vi "FTW-Endpoint-TCP-Connection-Get.vi"(8 "error in (no error)":errorcluster, 11 "FTW-Endpoint-TCP in":refnum<class "FTW-Endpoint-TCP.lvclass">) -> (0 "error out":errorcluster, 2 "Connection":refnum<k5>, 3 "FTW-Endpoint-TCP out":refnum<class "FTW-Endpoint-TCP.lvclass">)   [LabVIEW 2015, in "FTW-Endpoint-TCP.lvclass"]
uses:
  FTW-Endpoint-TCP.lvclass
  FTW-Endpoint-TCP.lvclass/FTW-Endpoint-TCP.ctl
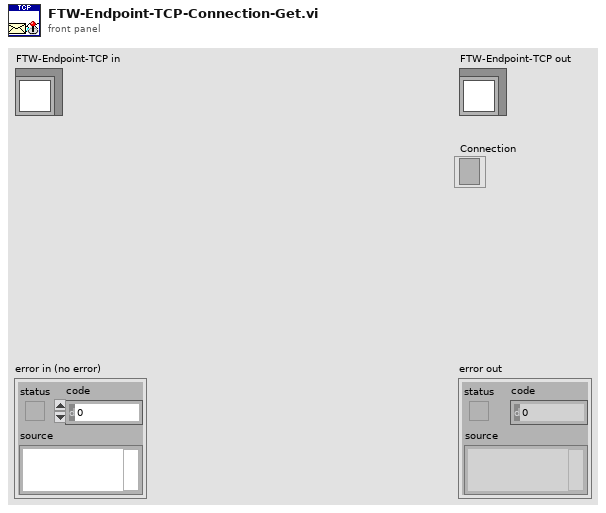
[diagram p1: front panel]
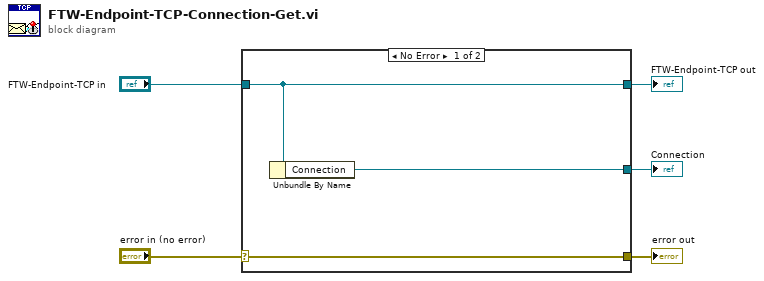
[diagram p0: block diagram]
diagram:
  n1 = case shown="No Error" "error in (no error)" {
    selector: "error in (no error)" -> [w8 w9]
    tunnel: [w8 w9] -> w4
    tunnel: [w7 w10] -> w2
    tunnel: "FTW-Endpoint-TCP in" -> [w7 w10]
    tunnel: [w6 _] -> w1
    frame No Error {
      n2 = Unbundle By Name(w7) -> ("Connection"=w6:refnum<k5>)
    }
    frame Error {
    }
  }
  "error out" <- w4
  "FTW-Endpoint-TCP out" <- w2
  "Connection" <- w1
